vi "NumericArrayToBoolArray.vi"(11 "InArray":dbl[](array[numeric])) -> (3 "OutArray":bool[](array[boolean]))   [LabVIEW 2019]
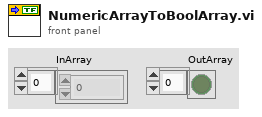
[diagram p1: front panel]
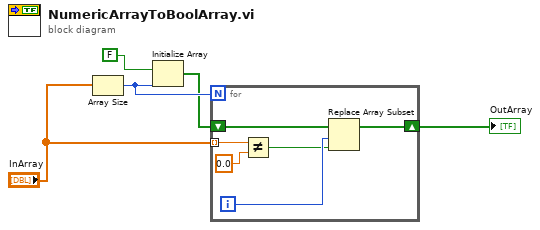
[diagram p0: block diagram]
diagram:
  n1 = Array Size(array="InArray") -> (size(s)=w4:i32)
  n2 = Initialize Array(FALSE, w4) -> (w2:bool[])
  n3 = for {
    N: w4 -> [_]
    tunnel: "InArray" -> [w9] mode=indexing
    shift-right: [w6] -> w1
    shift-left: w2 -> [w11]
    i -> [w10]
    n4 = Not Equal?(x=w9, y=0.0) -> (x != y?=w8:bool)
    n5 = Replace Array Subset(array=w11, new element=w8, index=w10) -> (w6:bool[])
  }
  "OutArray" <- w1
